vi "StreamWriter Strings.vi"() -> ()   [LabVIEW 2024, in "StreamWriter.lvlib" / "StreamWriter.lvclass"]
uses:
  StreamWriter.lvclass
panel:
  in  "Writer URL":string="Writer URL"
  in  "Buffer size":string="Buffer size"
  in  "Timeout":string="Timeout"
  in  "Select channels":string="Select channels"
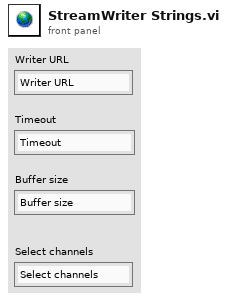
[diagram p1: front panel]
diagram:
